vi "Collate Provisional Visit Data.vi"(6 "DateTime":timestamp, 8 "Error In":errorcluster, 9 "Location":string, 10 "Line Items":T1[](array[typedef]) {"PriceIncDiscount (£)" format="%.2g"; "Discount(£)" format="%.2g"}, 11 "ReceiptImagePath":string) -> (0 "Error Out":errorcluster, 3 "Visits":T2 {"TotalSpend" format="£%.2g"; "SpendTaxedA" format="£%.2g"; "SpendTaxedB" format="£%.2g"})   [LabVIEW 2018, in "Main.lvlib"]
uses:
  Main.lvlib
  database/Visits--cluster.ctl
  ReceiptItemInfo.ctl
  database/Database.lvlib
  receipt parsing/Receipt Parsing.lvlib
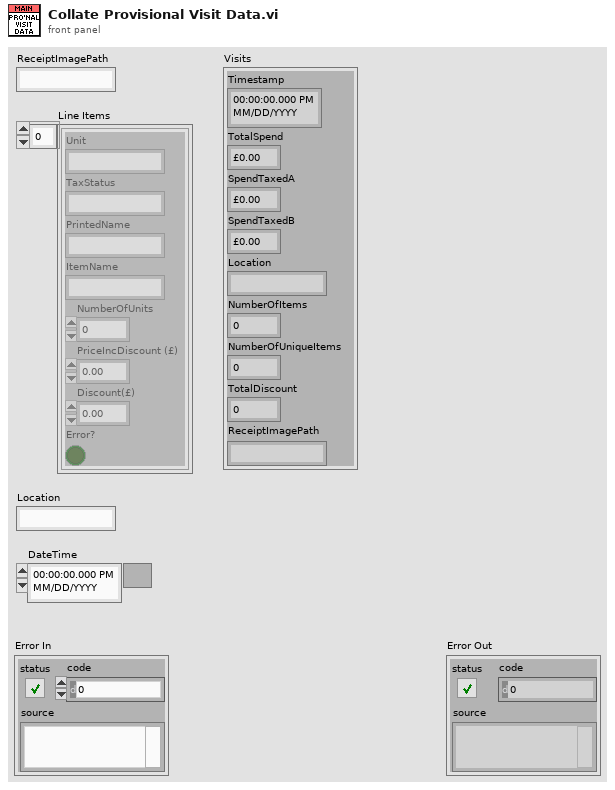
[diagram p1: front panel]
types:
  T1 = typedef "Receipt Parsing.lvlib/ReceiptItemInfo.ctl" = cluster{"Unit":string, "TaxStatus":string, "PrintedName":string, "ItemName":string, "NumberOfUnits":dbl, "PriceIncDiscount (£)":dbl, "Discount(£)":dbl, "Error?":bool}
  T2 = typedef "Database.lvlib/Visits--cluster.ctl" = cluster{"Timestamp":timestamp, "TotalSpend":dbl, "SpendTaxedA":dbl, "SpendTaxedB":dbl, "Location":string, "NumberOfItems":i32, "NumberOfUniqueItems":i32, "TotalDiscount":dbl, "ReceiptImagePath":string}
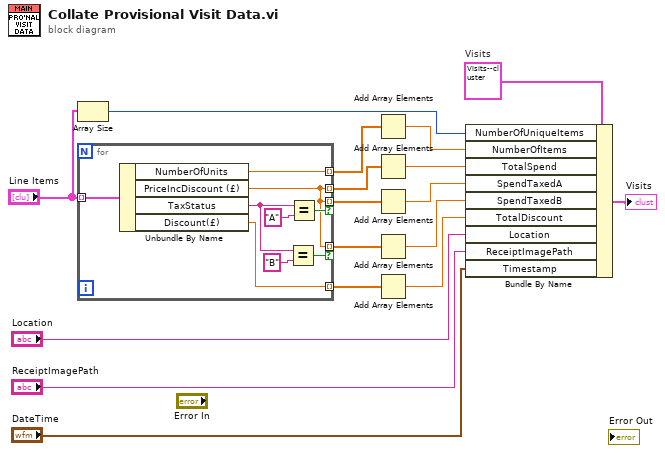
[diagram p0: block diagram]
diagram:
  w6 = T2 {"Timestamp"=timestamp(0 s since 1904-01-01), "TotalSpend"=0.0, "SpendTaxedA"=0.0, "SpendTaxedB"=0.0, "Location"="", "NumberOfItems"=0, "NumberOfUniqueItems"=0, "TotalDiscount"=0.0, "ReceiptImagePath"=""}  # Visits
  n1 = Array Size(array="Line Items") -> (size(s)=w7:i32)
  n2 = for {
    tunnel: "Line Items" -> [w26] mode=indexing
    tunnel: [w25] -> w3 mode=indexing
    tunnel: [w18] -> w1 mode=indexing if=w20
    tunnel: [w18] -> w2 mode=indexing if=w21
    tunnel: [w19] -> w4 mode=indexing
    tunnel: [w18] -> w5 mode=indexing
    n3 = Unbundle By Name(w26) -> ("NumberOfUnits"=w25:dbl, "PriceIncDiscount (£)"=w18:dbl, "TaxStatus"=w23:string, "Discount(£)"=w19:dbl)
    n4 = Equal?(x=w23, y="B") -> (x = y?=w21:bool)
    n5 = Equal?(x=w23, y="A") -> (x = y?=w20:bool)
  }
  n6 = Add Array Elements(numeric array=w3) -> (sum=w8:dbl)
  n7 = Add Array Elements(numeric array=w5) -> (sum=w9:dbl)
  n8 = Add Array Elements(numeric array=w1) -> (sum=w10:dbl)
  n9 = Add Array Elements(numeric array=w2) -> (sum=w11:dbl)
  n10 = Add Array Elements(numeric array=w4) -> (sum=w12:dbl)
  n11 = Bundle By Name(cluster=w6, "NumberOfUniqueItems"=w7, "NumberOfItems"=w8, "TotalSpend"=w9, "SpendTaxedA"=w10, "SpendTaxedB"=w11, "TotalDiscount"=w12, "Location"="Location", "ReceiptImagePath"="ReceiptImagePath", "Timestamp"="DateTime") -> (→"Visits":T2)
